vi "Command.vi"(8 "error in (no error)":errorcluster, 9 "arguments (none)":u32[](array[numeric]), 10 "command":string, 11 "Arinst SSA-TG in":refnum<class "PL Arinst SSA-TG.lvclass">) -> (0 "error out":errorcluster, 2 "response data":string, 3 "Arinst SSA-TG out":refnum<class "PL Arinst SSA-TG.lvclass">)   [LabVIEW 2015, in "PL Arinst SSA-TG.lvclass"]
doc: "Sends <b>command</b> with <b>command arguments</b> to device and returns <b>response data</b>."
uses:
  PL Arinst SSA-TG.lvclass
  PL Arinst SSA-TG.lvclass/PL Arinst SSA-TG.ctl
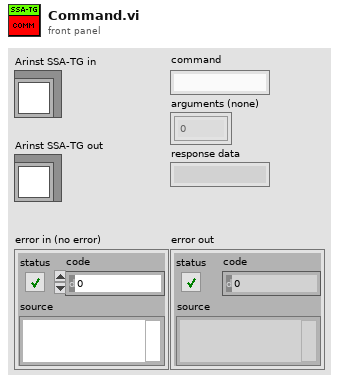
[diagram p1: front panel]
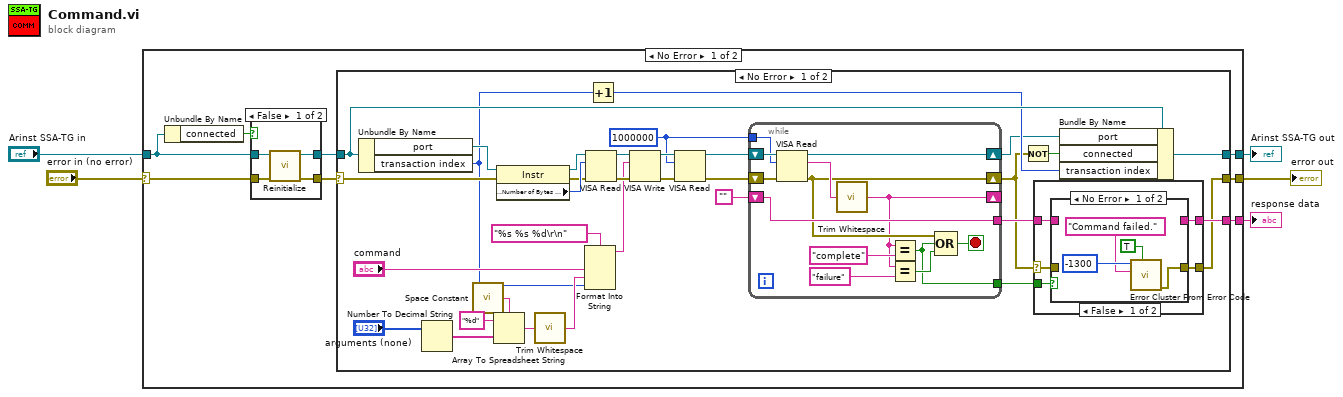
[diagram p0: block diagram]
diagram:
  n1 = case shown="No Error" "error in (no error)" {
    selector: "error in (no error)" -> [w11 w81]
    tunnel: "Arinst SSA-TG in" -> [w12 w80]
    tunnel: [w8 w81] -> w2
    tunnel: [w7 w80] -> w3
    tunnel: [w6 _] -> w1
    frame No Error {
      n2 = Unbundle By Name(w12) -> ("connected"=w13:bool)
      n3 = case shown="False" w13 {
        tunnel: w12 -> [w77 w79]
        tunnel: w11 -> [w76 w78]
        tunnel: [w75 w79] -> w9
        tunnel: [w74 w78] -> w10
        frame False {
          n4 = call "Reinitialize.vi"("error in (no error)"=w76, "Arinst SSA-TG in"=w77) -> ("error out"=w74:errorcluster, "Arinst SSA-TG out"=w75:refnum<class "PL Arinst SSA-TG.lvclass">)  [unwired: 8 in]
        }
        frame True {
        }
      }
      n5 = case shown="No Error" w10 {
        selector: w10 -> [w37 w73]
        tunnel: w9 -> [w44 w72]
        tunnel: [w14 w73] -> w8
        tunnel: [w34 w72] -> w7
        tunnel: [w15 _] -> w6
        frame No Error {
          w21 = u32 1000000 ("byte count")
          n6 = Unbundle By Name(w44) -> ("port"=w38:refnum<visa-resource-name>, "transaction index"=w25:u8)
          n7 = Number To Decimal String(number="arguments (none)") -> (decimal integer string=w28:string[])  [unwired: 1 in]
          n8 = call <vilib>:"Space Constant.vi"() -> ("String"=w29:string)
          n9 = Array To Spreadsheet String(delimiter (Tab)=w29, array=w28, 3:"%d" ("format string")) -> (spreadsheet string=w31:string)
          n10 = property class="Instr"(reference=w38, error in=w37) -> (reference out=w41:refnum<visa-resource-name>, error out=w36:errorcluster, "Serial Settings:Number of Bytes at Serial Port"=w42:u32)
          n11 = call <vilib>:"Trim Whitespace.vi"("string"=w31) -> ("trimmed string"=w26:string)  [unwired: 1 in]
          n12 = Format Into String(format string="%s %s %d\r\n", "command", w26, w25) -> (resulting string=w35:string)  [unwired: 2 in, 1 out]
          n13 = VISA Read(VISA resource name=w41, byte count=w42, error in (no error)=w36) -> (VISA resource name out=w40:refnum<visa-resource-name>, error out=w39:errorcluster)  [unwired: 2 out]
          n14 = Increment(x=w25) -> (x+1=w24:u8)
          n15 = VISA Write(VISA resource name=w40, write buffer=w35, error in (no error)=w39) -> (VISA resource name out=w46:refnum<visa-resource-name>, error out=w45:errorcluster)  [unwired: 1 out]
          n16 = VISA Read(VISA resource name=w46, byte count=w21, error in (no error)=w45) -> (VISA resource name out=w22:refnum<visa-resource-name>, error out=w23:errorcluster)  [unwired: 2 out]
          n17 = while {
            shift-right: [w65] -> w17
            shift-left: w23 -> [w71]
            shift-right: [w68] -> w20
            shift-left: w22 -> [w70]
            tunnel: w21 -> [w69]
            shift-right: [w59] -> _
            shift-left: "" -> [w67]
            tunnel: [w67] -> w18
            tunnel: [w60] -> w16
            stop <- w62 stop-if-true
            n18 = VISA Read(VISA resource name=w70, byte count=w69, error in (no error)=w71) -> (VISA resource name out=w68:refnum<visa-resource-name>, read buffer=w66:string, error out=w65:errorcluster)  [unwired: 1 out]
            n19 = call <vilib>:"Trim Whitespace.vi"("string"=w66) -> ("trimmed string"=w59:string)  [unwired: 1 in]
            n20 = Equal?(x=w59, y="complete") -> (x = y?=w60:bool)
            n21 = Equal?(x=w59, y="failure") -> (x = y?=w63:bool)
            n22 = Compound Arithmetic op=OR(w65, w60, w63) -> (w62:bool)
          }
          n23 = Not(x=w17) -> (.not. x?=w43:bool)
          n24 = case shown="No Error" w17 {
            selector: w17 -> [w48 w58]
            tunnel: w18 -> [w50 _]
            tunnel: w16 -> [w51 _]
            tunnel: [w49 _] -> w15
            tunnel: [w47 w58] -> w14
            frame No Error {
              n25 = case shown="False" w51 {
                tunnel: w50 -> [_ w57]
                tunnel: [_ w57] -> w49
                tunnel: w48 -> [_ w56]
                tunnel: [w52 w56] -> w47
                frame False {
                  n26 = call <vilib>:"Error Cluster From Error Code.vi"("show call chain? (False)"=TRUE, "error message (\"\")"="Command failed." ("format string"), "error code (0)"=-1300) -> ("error out"=w52:errorcluster)  [unwired: 6 in]
                }
                frame True {
                }
              }
            }
            frame Error {
            }
          }
          n27 = Bundle By Name(cluster=w44, "port"=w20, "connected"=w43, "transaction index"=w24) -> (w34:refnum<class "PL Arinst SSA-TG.lvclass">)
        }
        frame Error {
        }
      }
    }
    frame Error {
    }
  }
  "Arinst SSA-TG out" <- w3
  "error out" <- w2
  "response data" <- w1
